vi "Init.vi"(4 "Data Queue Names":string[](array[string]), 6 "Data Notifier Names":string[](array[string]), 7 "Name":string, 8 "error in (no error)":errorcluster, 10 "MSS":refnum<class "Measure and Stimulus Subsystems.lvclass">, 11 "Sample Temp PWM Control in":refnum<class "Sample Temp PWM Control.lvclass">) -> (0 "error out":errorcluster, 3 "Sample Temp PWM Control out":refnum<class "Sample Temp PWM Control.lvclass">)   [LabVIEW 2023, in "Sample Temp PWM Control.lvclass"]
uses:
  Sample Temp PWM Control.lvclass
  Measure and Stimulus Subsystems/Measure and Stimulus Subsystems.lvclass
  Task/Task Base/Task Base.lvclass
  Sample Temp PWM Control.lvclass/Sample Temp PWM Control.ctl
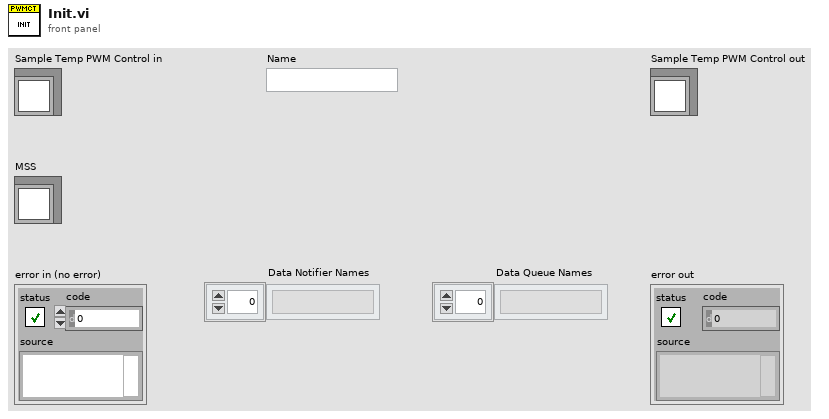
[diagram p1: front panel]
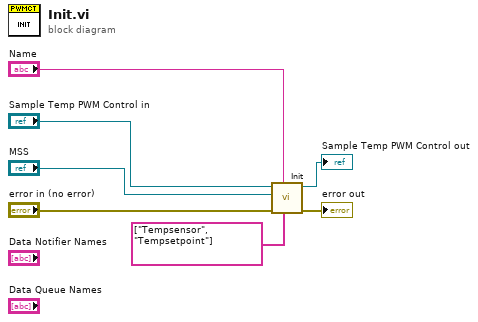
[diagram p0: block diagram]
diagram:
  n1 = call-parent "Init.vi"("Data Notifier Names"=string[] ["Tempsensor", "Tempsetpoint"], "Name"="Name", "error in (no error)"="error in (no error)", "MSS"="MSS", "Task Base in"="Sample Temp PWM Control in") -> ("error out"=→"error out":errorcluster, "Task Base out"=→"Sample Temp PWM Control out":refnum<class "Sample Temp PWM Control.lvclass">)  [unwired: 5 in]
